vi "Labview.vi"() -> ()   [LabVIEW 2018]
uses:
  Control 1.ctl
  System.Speech
panel:
  out "output":T1
  out "Outer loop Index":dbl
  in  "Braille letter Input":bool[][](array[boolean])=[[TRUE, FALSE, TRUE, TRUE, FALSE, FALSE], [TRUE, FALSE, FALSE, TRUE, FALSE, FALSE], [TRUE, FALSE, TRUE, FALSE, TRUE, FALSE], [TRUE, FALSE, TRUE, FALSE, TRUE, FALSE], [TRUE, FALSE, FALSE, TRUE, TRUE, FALSE]]
  in  "Array 4":bool[][](array[boolean])=[[TRUE, FALSE, FALSE, FALSE, FALSE, FALSE], [TRUE, FALSE, TRUE, FALSE, FALSE, FALSE], [TRUE, TRUE, FALSE, FALSE, FALSE, FALSE], [TRUE, TRUE, FALSE, TRUE, FALSE, FALSE], [TRUE, FALSE, FALSE, TRUE, FALSE, FALSE], [TRUE, TRUE, TRUE, FALSE, FALSE, FALSE], [TRUE, TRUE, TRUE, TRUE, FALSE, FALSE], [TRUE, FALSE, TRUE, TRUE, FALSE, FALSE], [FALSE, TRUE, TRUE, FALSE, FALSE, FALSE], [FALSE, TRUE, TRUE, TRUE, FALSE, FALSE], [TRUE, FALSE, FALSE, FALSE, TRUE, FALSE], [TRUE, FALSE, TRUE, FALSE, TRUE, FALSE], [TRUE, TRUE, FALSE, FALSE, TRUE, FALSE], [TRUE, TRUE, FALSE, TRUE, TRUE, FALSE], [TRUE, FALSE, FALSE, TRUE, TRUE, FALSE], [TRUE, TRUE, TRUE, FALSE, TRUE, FALSE], [TRUE, TRUE, TRUE, TRUE, TRUE, FALSE], [TRUE, FALSE, TRUE, TRUE, TRUE, FALSE], [FALSE, TRUE, TRUE, FALSE, TRUE, FALSE], [FALSE, TRUE, TRUE, TRUE, TRUE, FALSE], [TRUE, FALSE, FALSE, FALSE, TRUE, TRUE], [TRUE, FALSE, TRUE, FALSE, TRUE, TRUE], [FALSE, TRUE, TRUE, TRUE, FALSE, TRUE], [TRUE, TRUE, FALSE, FALSE, TRUE, TRUE], [TRUE, TRUE, FALSE, TRUE, TRUE, TRUE], [TRUE, FALSE, FALSE, TRUE, TRUE, TRUE], [FALSE, FALSE, FALSE, FALSE, FALSE, FALSE]]
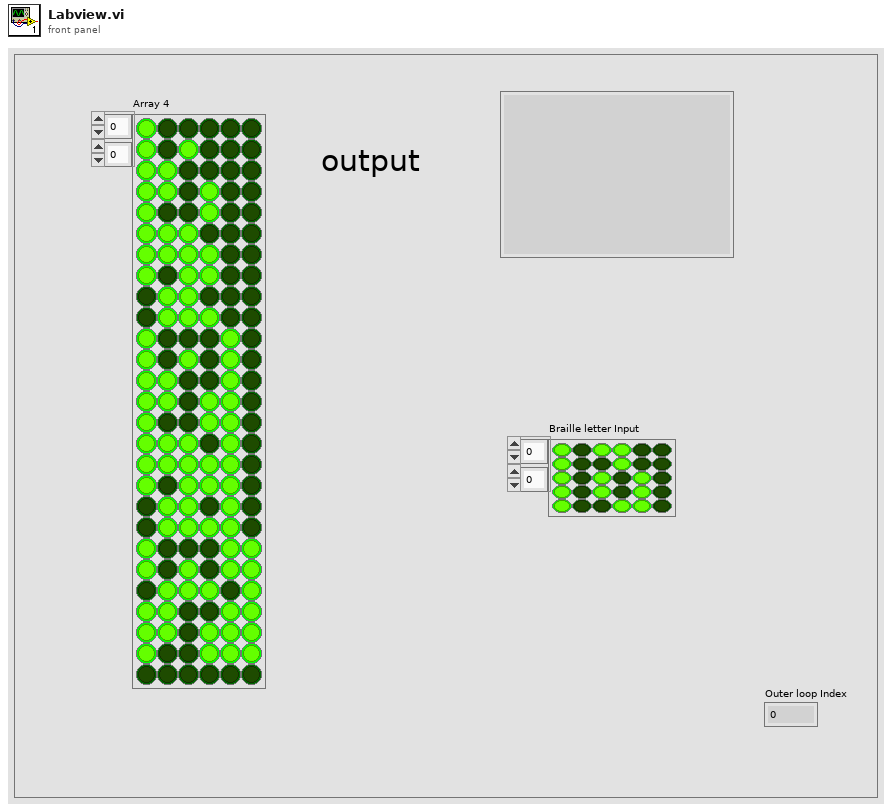
[diagram p1: front panel]
types:
  T1 = typedef "Control 1.ctl" = string
  T2 = typedef "Control 1" = string
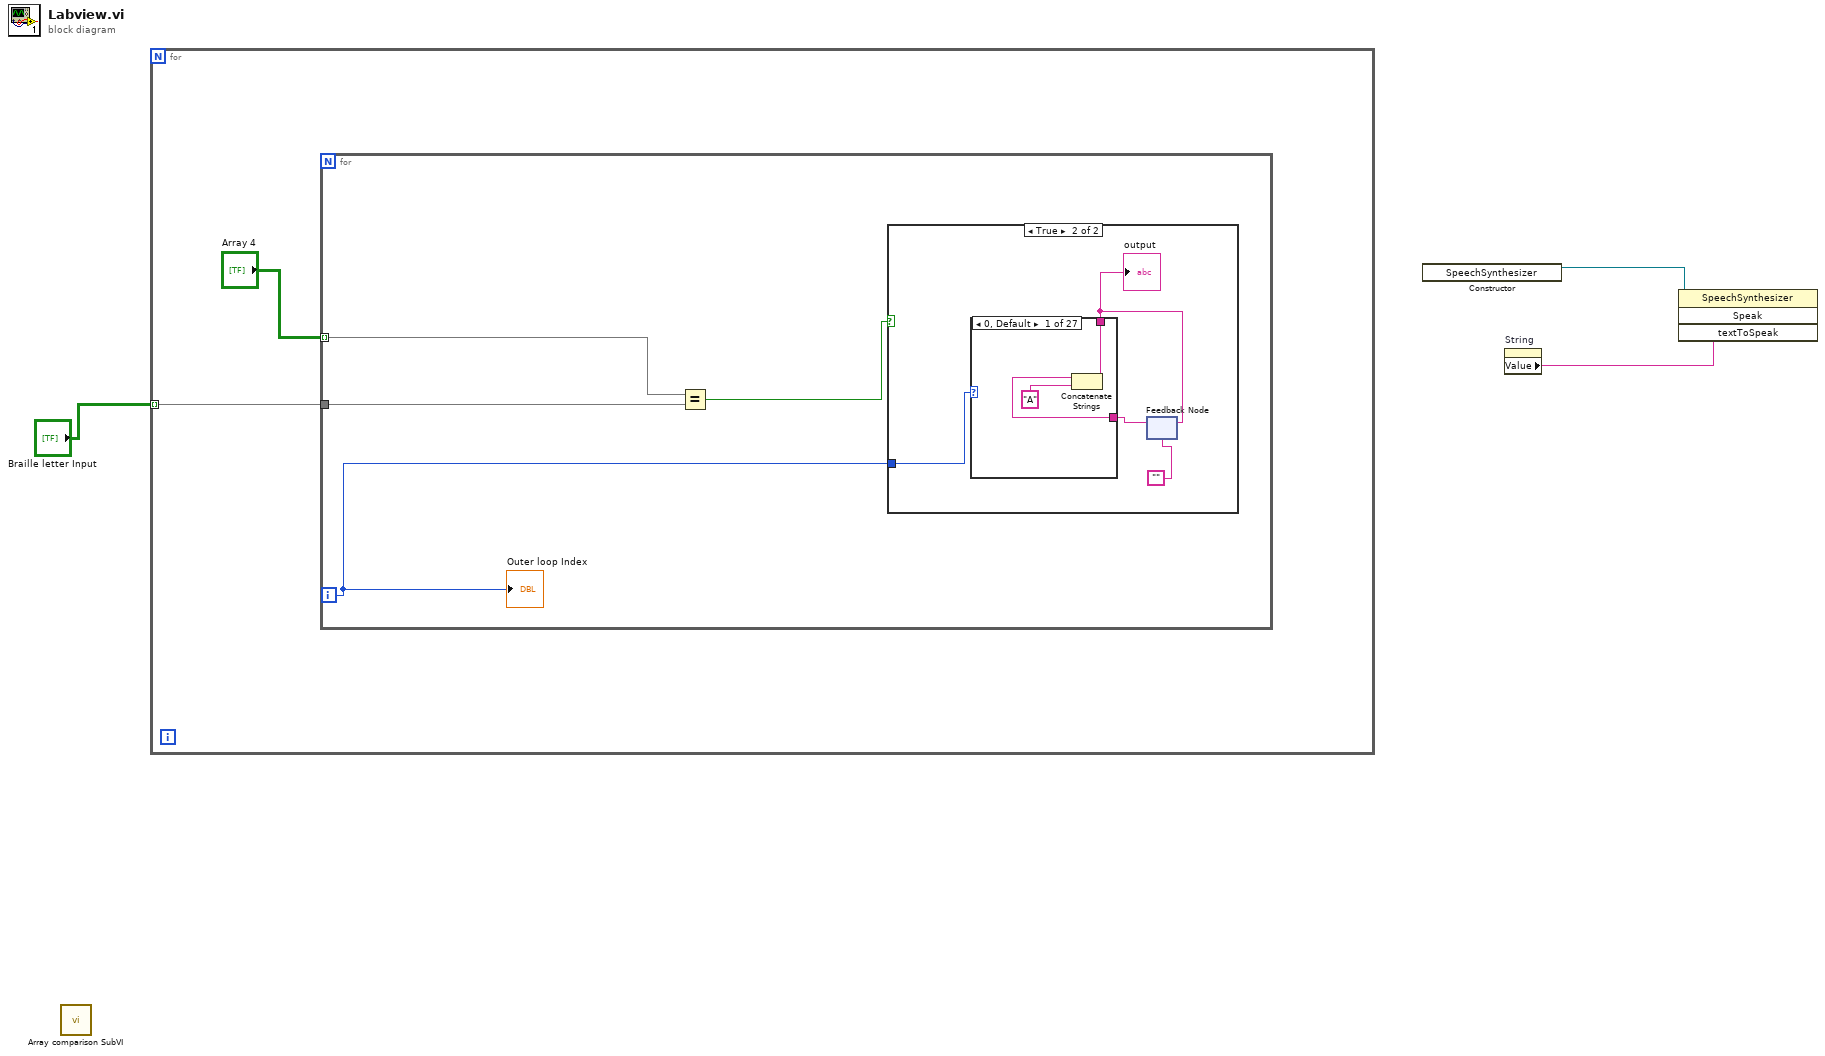
[diagram p0: block diagram]
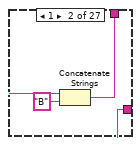
[diagram p3: hidden frame]
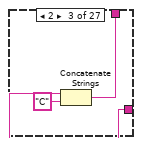
[diagram p4: hidden frame]
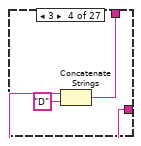
[diagram p5: hidden frame]
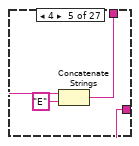
[diagram p6: hidden frame]
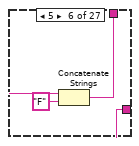
[diagram p7: hidden frame]
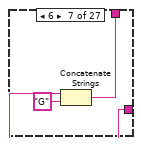
[diagram p8: hidden frame]
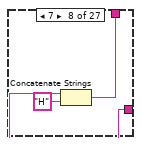
[diagram p9: hidden frame]
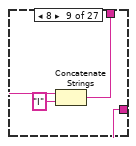
[diagram p10: hidden frame]
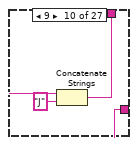
[diagram p11: hidden frame]
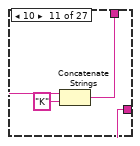
[diagram p12: hidden frame]
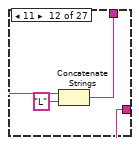
[diagram p13: hidden frame]
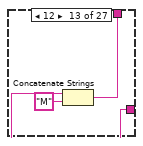
[diagram p14: hidden frame]
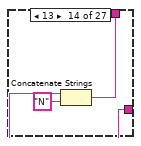
[diagram p15: hidden frame]
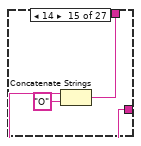
[diagram p16: hidden frame]
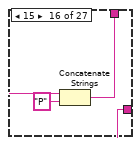
[diagram p17: hidden frame]
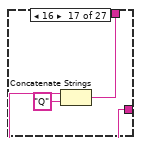
[diagram p18: hidden frame]
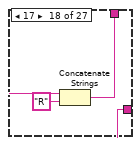
[diagram p19: hidden frame]
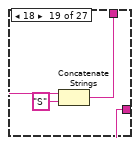
[diagram p20: hidden frame]
diagram:
  n1 = call "Array comparison SubVI.vi"() -> ()  [unwired: 11 in, 1 out]
  n2 = for {
    tunnel: "Braille letter Input" -> [w4] mode=indexing
    n3 = for {
      tunnel: "Array 4" -> [w7] mode=indexing
      tunnel: w4 -> [w6]
      i -> [w9]
      n4 = Equal?(x=w7, y=w6) -> (x = y?=w8:bool)
      n5 = case shown="True" w8 {
        tunnel: w9 -> [_ w11]
        frame False {
        }
        frame True {
          n6 = feedback #1("") -> (w13:string)
          n7 = case shown="0, Default" w11 {
            tunnel: [w16 w19 w22 w25 w28 w31 w34 w37 w40 w43 w46 w49 w52 w55 w58 w61 w64 w67 w70 w73 w76 w79 w82 w85 w88 w91 w94] -> w10
            tunnel: w13 -> [w15 w18 w21 w24 w27 w30 w33 w36 w39 w42 w45 w48 w51 w54 w57 w60 w63 w66 w69 w72 w75 w78 w81 w84 w87 w90 w93]
            frame 0, Default {
              n8 = Concatenate Strings(w15, "A") -> (w16:string)
            }
            frame 1 {
              n9 = Concatenate Strings(w18, "B" ("string")) -> (w19:string)
            }
            frame 2 {
              n10 = Concatenate Strings(w21, "C" ("string")) -> (w22:string)
            }
            frame 3 {
              n11 = Concatenate Strings(w24, "D" ("string")) -> (w25:string)
            }
            frame 4 {
              n12 = Concatenate Strings(w27, "E" ("string")) -> (w28:string)
            }
            frame 5 {
              n13 = Concatenate Strings(w30, "F" ("string")) -> (w31:string)
            }
            frame 6 {
              n14 = Concatenate Strings(w33, "G" ("string")) -> (w34:string)
            }
            frame 7 {
              n15 = Concatenate Strings(w36, "H" ("string")) -> (w37:string)
            }
            frame 8 {
              n16 = Concatenate Strings(w39, "I" ("string")) -> (w40:string)
            }
            frame 9 {
              n17 = Concatenate Strings(w42, "J" ("string")) -> (w43:string)
            }
            frame 10 {
              n18 = Concatenate Strings(w45, "K" ("string")) -> (w46:string)
            }
            frame 11 {
              n19 = Concatenate Strings(w48, "L" ("string")) -> (w49:string)
            }
            frame 12 {
              n20 = Concatenate Strings(w51, "M" ("string")) -> (w52:string)
            }
            frame 13 {
              n21 = Concatenate Strings(w54, "N" ("string")) -> (w55:string)
            }
            frame 14 {
              n22 = Concatenate Strings(w57, "O" ("string")) -> (w58:string)
            }
            frame 15 {
              n23 = Concatenate Strings(w60, "P" ("string")) -> (w61:string)
            }
            frame 16 {
              n24 = Concatenate Strings(w63, "Q" ("string")) -> (w64:string)
            }
            frame 17 {
              n25 = Concatenate Strings(w66, "R" ("string")) -> (w67:string)
            }
            frame 18 {
              n26 = Concatenate Strings(w69, "S" ("string")) -> (w70:string)
            }
            frame 19 {
              n27 = Concatenate Strings(w72, "T" ("string")) -> (w73:string)
            }
            frame 20 {
              n28 = Concatenate Strings(w75, "U" ("string")) -> (w76:string)
            }
            frame 21 {
              n29 = Concatenate Strings(w78, "V" ("string")) -> (w79:string)
            }
            frame 22 {
              n30 = Concatenate Strings(w81, "W" ("string")) -> (w82:string)
            }
            frame 23 {
              n31 = Concatenate Strings(w84, "X" ("string")) -> (w85:string)
            }
            frame 24 {
              n32 = Concatenate Strings(w87, "Y" ("string")) -> (w88:string)
            }
            frame 25 {
              n33 = Concatenate Strings(w90, "Z" ("string")) -> (w91:string)
            }
            frame 26 {
              n34 = Concatenate Strings(w93, "  " ("string")) -> (w94:string)
            }
          }
          "output" <- w10
          n35 = feedback-in #1(w10) -> ()
        }
      }
      "Outer loop Index" <- w9
    }
  }
  n36 = constructor class="SpeechSynthesizer"() -> (reference out=w2:refnum<k24>)  [unwired: 3 in, 2 out]
  n37 = property on="String" class="Str (strict)"() -> ("Value"=w1:T2)  [unwired: 2 in, 2 out]
  n38 = invoke class="SpeechSynthesizer" method="Speak"(reference=w2, "textToSpeak"=w1) -> ()  [unwired: 2 in, 4 out]
